vi "ソース コード.vi"() -> ()   [LabVIEW 2014]
panel:
  out "x+y":dbl
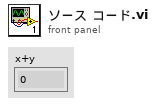
[diagram p1: front panel]
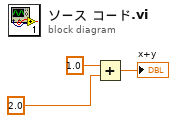
[diagram p0: block diagram]
diagram:
  n1 = Add(x=1.0, y=2.0) -> (x+y=→"x+y":dbl)
